vi "Set Panel View.lvclass.vi"(8 "error in (no error)":errorcluster, 10 "Panel View.lvclass":refnum<class "Panel View.lvclass">, 11 "Panel Manager Controller.lvclass":refnum<class "Panel Manager Controller.lvclass">) -> (0 "error out":errorcluster, 3 "Panel Manager Controller.lvclass out":refnum<class "Panel Manager Controller.lvclass">)   [LabVIEW 2015, in "Panel Manager Controller.lvclass"]
uses:
  Panel Manager Controller.lvclass
  Panel View/Panel View.lvclass
  Panel Manager Controller.lvclass/Panel Manager Controller.ctl
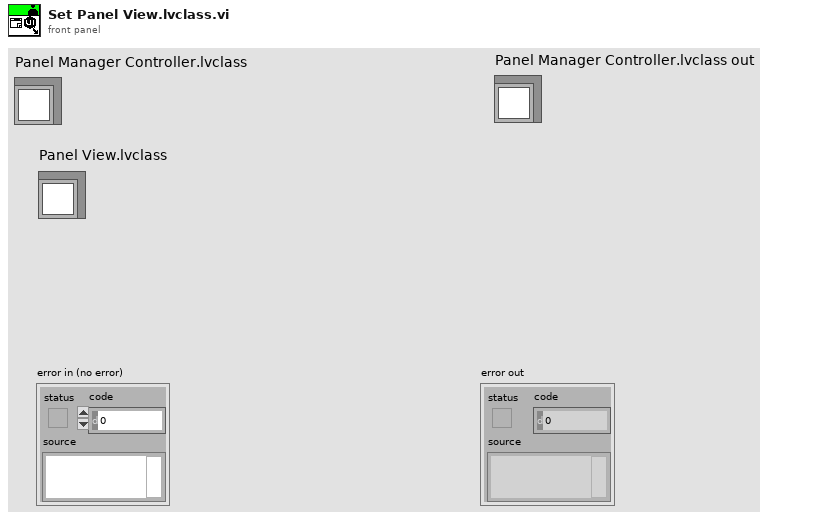
[diagram p1: front panel]
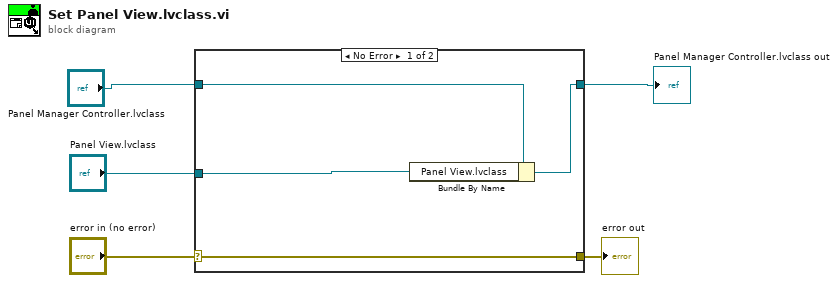
[diagram p0: block diagram]
diagram:
  n1 = case shown="No Error" "error in (no error)" {
    selector: "error in (no error)" -> [w9 w10]
    tunnel: [w9 w10] -> w4
    tunnel: [w7 w11] -> w1
    tunnel: "Panel Manager Controller.lvclass" -> [w8 w11]
    tunnel: "Panel View.lvclass" -> [w6 _]
    frame No Error {
      n2 = Bundle By Name(cluster=w8, "Panel View.lvclass"=w6) -> (w7:refnum<class "Panel Manager Controller.lvclass">)
    }
    frame Error {
    }
  }
  "error out" <- w4
  "Panel Manager Controller.lvclass out" <- w1
